vi "Pfeiffer-RVC300.key lock.vi"(0 "i ref in":refnum<vi>, 2 "Lock?":bool=TRUE, 5 "error in (no error)":errorcluster) -> (14 "i ref out":refnum<vi>, 16 "key_status":string, 19 "error out":errorcluster)   [LabVIEW 2014, in "Pfeiffer-RVC300.lvlib"]
doc: "This is the constructor of a class.\n\nLicense Agreement for this software:\n\nCopyright (C)\nGesellschaft für Schwerionenforschung, GSI\nPlanckstr. 1\n64291 Darmstadt\nGermany\n\nContact: D.Beck@gsi.de \n\nThis program is free software; you can redistribute it and/or modify it under the terms of the \nGNU General Public License as published by the Free Software Foundation; either version 2 of \nthe license, or (at your option) any later version.\n\nThis program is distributed in the hope that it will be useful, but WITHOUT ANY WARRANTY; \nwithout even the implied warranty of MERCHANTABILITY or FITNESS FOR A PARTICULAR PURPOSE. See the GNU General License for more details (http://www.gnu.org).\n\nGesellschaft für Schwerionenforschung, GSI\nPlanckstr. 1, 64291 Darmstadt, Germany\nFor all questions and ideas contact: M.Richter@gsi.de, H.Brand@gsi.de or D.Beck@gsi.de.\nLast update: 16-JUN-2004"
uses:
  Pfeiffer-RVC300.lvlib
  CS_Core/CSSystem/CoreDefs/CoreDefs.error_type.ctl
  instr.lib/RVC300/RVC-300.lvlib
  CS_Core/CSSystem/CoreLib/CoreLib.lvlib
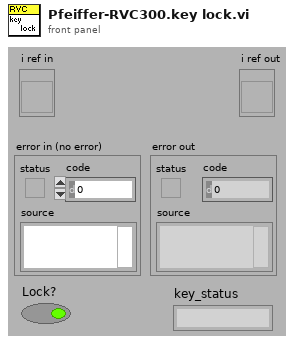
[diagram p1: front panel]
types:
  T1 = typedef "CoreDefs.error_type.ctl" = enum16{"no error", "can't load process", "can't unload process", "process does not exist", "can't install process", "can't remove process", "unknown function", "time out", "can't execute function", "duplicate queue name", "super not found", "caller queue invalid", "can't ping process", "unknown error", "VISA Error", "VISA timeout", "GPIB timeout", "GPIB error", "communication error", "data type mismatch", "can't read data from OPC server", "can't write data to OPC server", "OET error", "function not implemented", "process already exists", "invalid Shared Variable name", "error writing Shared Variable", "error reading Shared Variable", "invalid client name", "corrupt database", "unknown class", "call not authorized", "parameter out of range", "OET timeout: can't get data to modify", "invalid queue name", "requested operation incompatible with current state", "event undefined", "event disabled", "state undefined", "caller is not a friend", "EventBuilder: bad eventID", "EventBuilder: no DAQ devices", "a thread must not stop itself", "UNUSED ELEMENT4", "DiscArchiver: eventData incomplete", "DiscArchiver: eventData does not belong to run", "DiscArchiver: can't open file", "DiscArchiver: can't write to file", "DiscArchiver: available disc space low", "can't acquire semaphore", "error reading data from database", "notifier object is not existing", "can't register process", "can't unregister process", "illegal event type", "object disabled", "object already exists", "can't change state", "Instrument not found", "no connection to remote node", "invalid reference", "N/A", "UNUSED ELEMENT 1", "element not found", "illegal TCP/IP connection detected", "object does not exist", "invalid access ID", "unknown CS system", "invalid privilige", "unsupported data type", "unsupported server type", "IO server already exists", "Shared Variable already exists"}
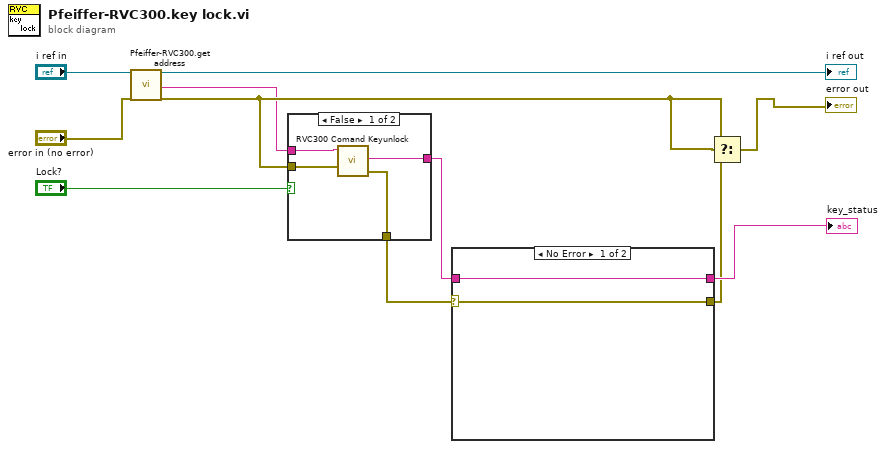
[diagram p0: block diagram]
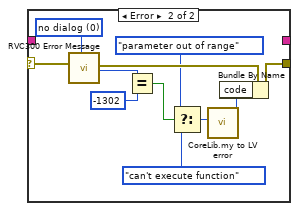
[diagram p2: hidden frame]
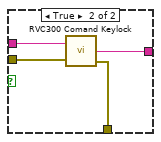
[diagram p3: hidden frame]
diagram:
  n1 = call "Pfeiffer-RVC300.get address.vi"("i ref in"="i ref in", "error in (no error)"="error in (no error)") -> ("i ref out"=→"i ref out":refnum<vi>, "address"=w6:string, "error out"=w7:errorcluster)  [unwired: 15 in]
  n2 = case shown="False" "Lock?" {
    tunnel: w6 -> [w15 w19]
    tunnel: w7 -> [w14 w18]
    tunnel: [w13 w17] -> w2
    tunnel: [w12 w16] -> w3
    frame False {
      n3 = call "RVC300 Comand Keyunlock.vi"("RVC300 VISA Resource Name"=w15, "error in (no error)"=w14) -> ("RVC Key status"=w13:string, "error out"=w12:errorcluster)  [unwired: 1 out]
    }
    frame True {
      n4 = call "RVC300 Comand Keylock.vi"("RVC300 VISA Resource Name"=w19, "error in (no error)"=w18) -> ("RVC Key status"=w17:string, "error out"=w16:errorcluster)  [unwired: 1 out]
    }
  }
  n5 = case shown="No Error" w3 {
    selector: w3 -> [w21 w32]
    tunnel: [w21 w29] -> w1
    tunnel: w2 -> [w20 _]
    tunnel: [w20 _] -> w5
    frame No Error {
    }
    frame Error {
      w28 = u16 0 items=["no dialog", "OK message", "continue or stop message"] ("type of dialog (OK msg:1)")
      n6 = call "RVC300 Error Message.vi"("error in (no error)"=w32, "type of dialog (OK msg:1)"=w28) -> ("error out"=w31:errorcluster, "code out"=w27:i32)  [unwired: 12 in, 4 out]
      n7 = Equal?(x=w27, y=-1302) -> (x = y?=w25:bool)
      n8 = Select(t=CoreDefs.error_type."parameter out of range" ("ErrorTypes"), s=w25, f=CoreDefs.error_type."can't execute function" ("ErrorTypes")) -> (s? t:f=w22:T1)
      n9 = call "CoreLib.my to LV error.vi"("ErrorTypes"=w22) -> ("LV error code"=w30:i32)  [unwired: 17 in, 1 out]
      n10 = Bundle By Name(cluster=w31, "code"=w30) -> (w29:errorcluster)
    }
  }
  "key_status" <- w5
  n11 = Select(t=w7, s=w7, f=w1) -> (s? t:f=→"error out":errorcluster)
